vi "ArrangeNodes ConvertNodeDataToBounds.vi"(1 "NodeData":T1 {"maxCornerDist" format="%.2f"; "h" format="%.2f"; "w" format="%.2f"; "dy" format="%.2f"; "dx" format="%.2f"; "y" format="%.2f"; "x" format="%.2f"}) -> (0 "NodeBounds":cluster{"x":dbl, "y":dbl, "w":dbl, "h":dbl})   [LabVIEW 2020]
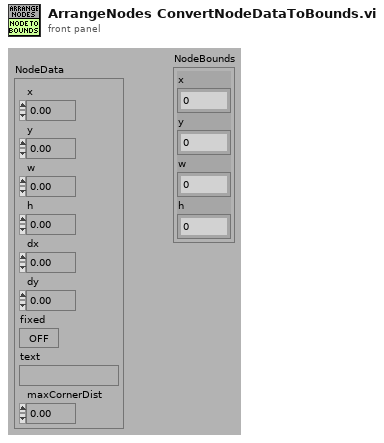
[diagram p1: front panel]
types:
  T1 = cluster{"x":dbl, "y":dbl, "w":dbl, "h":dbl, "dx":dbl, "dy":dbl, "fixed":bool, "text":string, "maxCornerDist":dbl}
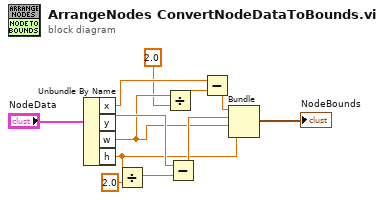
[diagram p0: block diagram]
diagram:
  n1 = Unbundle By Name("NodeData") -> ("x"=w7:dbl, "y"=w11:dbl, "w"=w5:dbl, "h"=w10:dbl)
  n2 = Divide(x=w10, y=2.0) -> (x/y=w3:dbl)
  n3 = Divide(x=w5, y=2.0) -> (x/y=w6:dbl)
  n4 = Subtract(x=w11, y=w3) -> (x-y=w12:dbl)
  n5 = Subtract(x=w7, y=w6) -> (x-y=w8:dbl)
  n6 = Bundle(w8, w12, "w"=w5, "h"=w10) -> (→"NodeBounds":cluster{dbl, dbl, "w":dbl, "h":dbl})  [unwired: 1 out]
